vi "New Message Command (RT-RT).vi"(6 "monitor(F)":bool, 8 "error in":errorcluster, 9 "Message Command Configuration":T1, 10 "messageBufferIDRef":i32, 11 "name":string) -> (0 "error out":errorcluster, 2 "Message Command ID out":i32, 3 "new message command":refnum<k24>)   [LabVIEW 2020, in "Ballard_1553_Hardware_ni.lvlib"]
uses:
  Ballard_1553_Hardware_ni.lvlib
  C:/Users/Administrator/Desktop/GIT/Ballard-MIL-STD-1553-Custom-Device/Source/System Explorer/SubVIs/Parse XML Ballard/1.2/BTIXML_SerDes.dll
  Ballard-MIL-STD-1553-Custom-Device/Source/System Explorer/SubVIs/Parse XML Ballard/1.2/BTIXML_SerDes.dll
  _typedefs/MessageCommand_RTRT_type.ctl
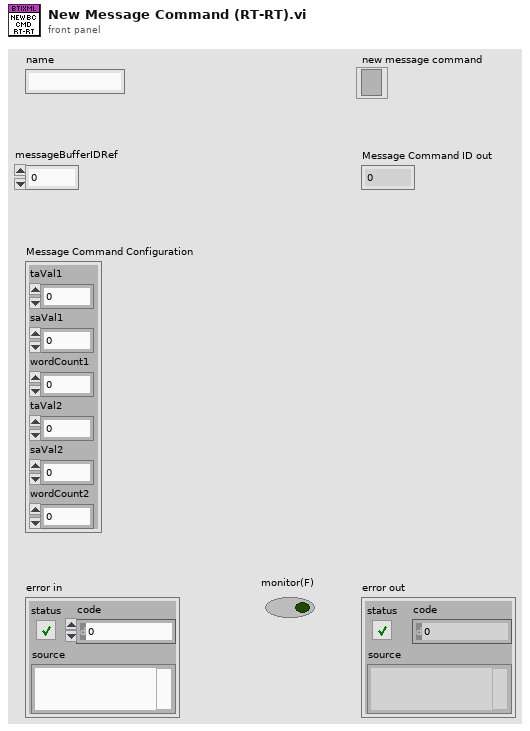
[diagram p1: front panel]
types:
  T1 = typedef "Ballard_1553_Hardware_ni.lvlib/MessageCommand_RTRT_type.ctl" = cluster{"taVal1":i8, "saVal1":i8, "wordCount1":i8, "taVal2":i8, "saVal2":i8, "wordCount2":i8}
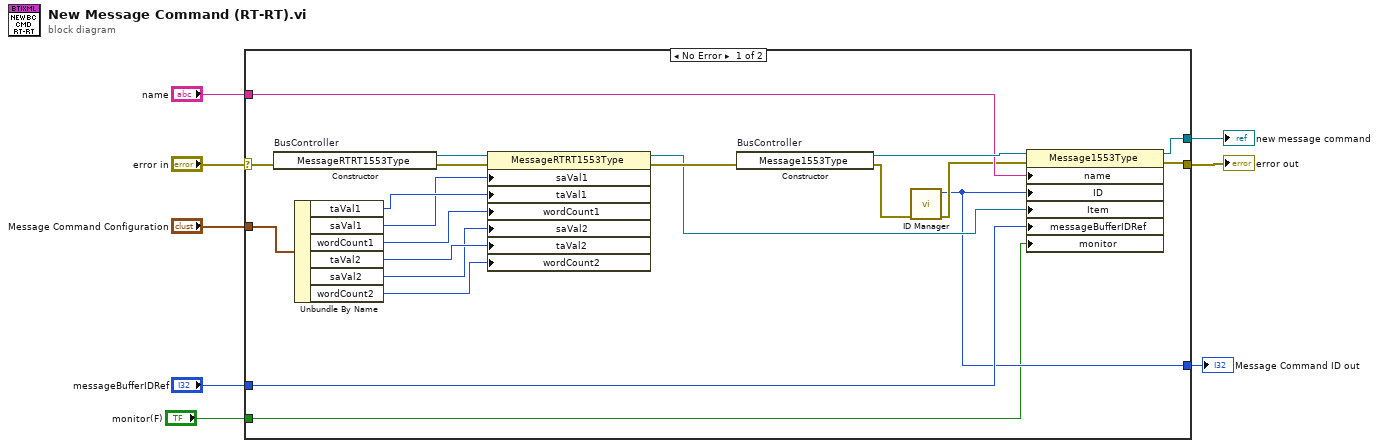
[diagram p0: block diagram]
diagram:
  n1 = case shown="No Error" "error in" {
    selector: "error in" -> [w29 w30]
    tunnel: [w20 w30] -> w7
    tunnel: "name" -> [w23 _]
    tunnel: "messageBufferIDRef" -> [w21 _]
    tunnel: [w19 _] -> w4
    tunnel: "Message Command Configuration" -> [w18 _]
    tunnel: [w13 _] -> w2
    tunnel: "monitor(F)" -> [w9 _]
    frame No Error {
      n2 = constructor on="BusController" class="MessageRTRT1553Type"(error in=w29) -> (reference out=w28:refnum<k24>, error out=w27:errorcluster)  [unwired: 2 in, 1 out]
      n3 = Unbundle By Name(w18) -> ("taVal1"=w17:i8, "saVal1"=w16:i8, "wordCount1"=w15:i8, "taVal2"=w12:i8, "saVal2"=w11:i8, "wordCount2"=w10:i8)
      n4 = property class="MessageRTRT1553Type"(reference=w28, error in=w27, "saVal1"=w16, "taVal1"=w17, "wordCount1"=w15, "saVal2"=w11, "taVal2"=w12, "wordCount2"=w10) -> (reference out=w14:refnum<k24>, error out=w25:errorcluster)
      n5 = constructor on="BusController" class="Message1553Type"(error in=w25) -> (reference out=w26:refnum<k24>, error out=w24:errorcluster)  [unwired: 2 in, 1 out]
      n6 = call "ID Manager.vi"("error in"=w24) -> ("error out"=w22:errorcluster, "ID out"=w13:i32)  [unwired: 9 in]
      n7 = property class="Message1553Type"(reference=w26, error in=w22, "name"=w23, "ID"=w13, "Item"=w14, "messageBufferIDRef"=w21, "monitor"=w9) -> (reference out=w19:refnum<k24>, error out=w20:errorcluster)
    }
    frame Error {
    }
  }
  "error out" <- w7
  "new message command" <- w4
  "Message Command ID out" <- w2
